vi "Create SystemLink Feed.vi"(0 "SystemLink repo in":T1, 5 "feed name":string, 7 "feed description":string, 9 "timeout (ms) (10000)":u32=10000, 11 "error in (no error)":errorcluster) -> (4 "SystemLink repo out":T1, 6 "feed name out":string, 10 "timed out?":bool, 15 "error out":errorcluster)   [LabVIEW 2017, in "SystemLink_Repo_API.lvlib"]
doc: "Creates a new feed in the SystemLink repository."
uses:
  SystemLink_Repo_API.lvlib
  <vilib>/JDP Science/JSONtext/LVClass Serializer/JSONtext LVClass Serializer.lvclass
  <vilib>/httpClient/LabVIEWHTTPClient.lvlib
  11e22a70-f141-46f2-99f4-c1a96e6a99a8.vi
  <vilib>/httpClient/POSTBuffer.vi
  <vilib>/httpClient/ClientHandle.ctl
  _support/systemlink repo.ctl
panel:
  out "job ID":string
  out "body":string
  out "headers":string
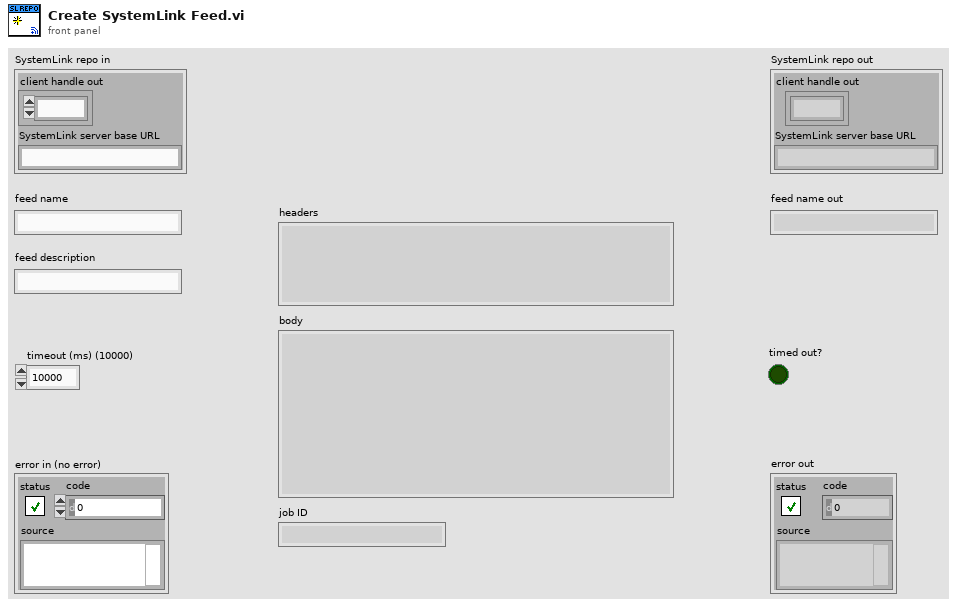
[diagram p1: front panel]
types:
  T1 = typedef "SystemLink_Repo_API.lvlib/systemlink repo.ctl" = cluster{"client handle out":T2, "SystemLink server base URL":string}
  T2 = typedef "LabVIEWHTTPClient.lvlib/ClientHandle.ctl" = refnum<k1>
  T3 = cluster{"feedName":string, "description":string, "platform":string}
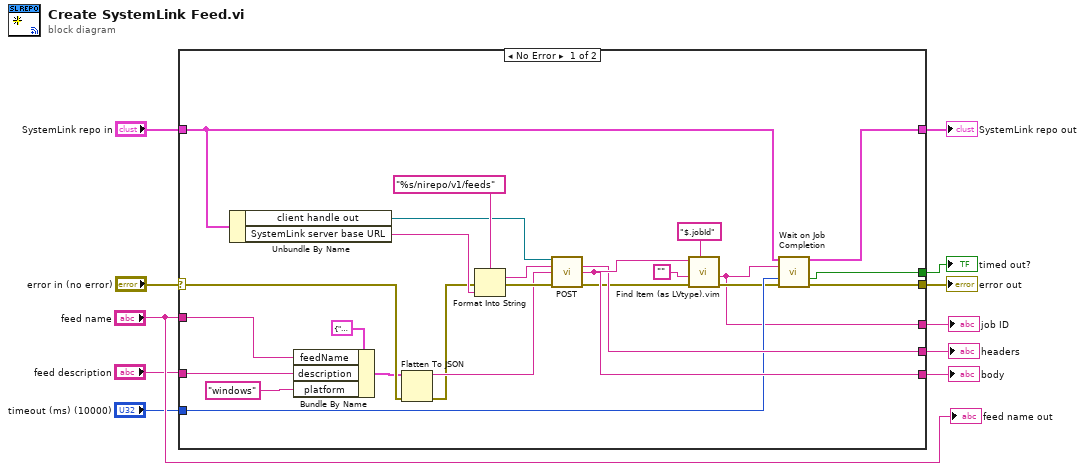
[diagram p0: block diagram]
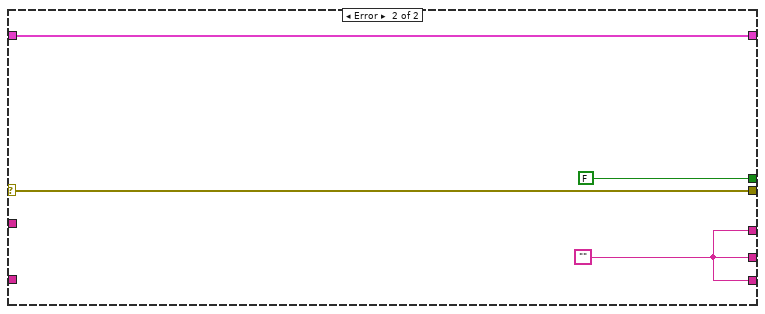
[diagram p2: hidden frame]
diagram:
  n1 = case shown="No Error" "error in (no error)" {
    selector: "error in (no error)" -> [w30 w40]
    tunnel: "SystemLink repo in" -> [w29 w39]
    tunnel: [w34 w40] -> w9
    tunnel: [w36 w37] -> w8
    tunnel: [w35 w37] -> w7
    tunnel: [w33 w39] -> w6
    tunnel: "feed name" -> [w16 _]
    tunnel: "feed description" -> [w14 _]
    tunnel: "timeout (ms) (10000)" -> [w32 _]
    tunnel: [w31 FALSE ("timed out?")] -> w3
    tunnel: [w17 w37] -> w2
    frame No Error {
      n2 = Unbundle By Name(w29) -> ("client handle out"=w26:T2, "SystemLink server base URL"=w22:string)
      n3 = Bundle By Name(cluster=T3 {"feedName"="", "description"="", "platform"=""}, "feedName"=w16, "description"=w14, "platform"="windows") -> (w13:T3)
      n4 = Flatten To JSON(anything=w13, error in (no error)=w30) -> (JSON string=w21:string, 11:w20:errorcluster)  [unwired: 1 in]
      n5 = Format Into String(format string="%s/nirepo/v1/feeds", error in=w20, w22) -> (resulting string=w27:string, error out=w25:errorcluster)  [unwired: 1 in]
      n6 = call-poly <vilib>:"POST.vi"("client handle"=w26, "url"=w27, "buffer"=w21, "error in (no error)"=w25) -> ("headers"=w35:string, "body"=w36:string, "error out"=w19:errorcluster)  [unwired: 8 in, 1 out]
      n7 = call "Find Item (as LVtype).vim"("$Path or Item Name"="$.jobId", "error in (no error)"=w19, "Data Type and Default Value"="", "JSON"=w36) -> ("error out"=w18:errorcluster, "Data"=w17:string)  [unwired: 4 in, 2 out]
      n8 = call "Wait on Job Completion.vi"("SystemLink repo in"=w29, "job ID"=w17, "timeout (ms) (10000)"=w32, "error in (no error)"=w18) -> ("SystemLink repo out"=w33:T1, "timed out?"=w31:bool, "error out"=w34:errorcluster)  [unwired: 8 in, 1 out]
    }
    frame Error {
      w37 = "" ("headers")
    }
  }
  "error out" <- w9
  "SystemLink repo out" <- w6
  "headers" <- w7
  "body" <- w8
  "timed out?" <- w3
  "job ID" <- w2
  "feed name out" <- "feed name"
